vi "Write Classes.vi"(8 "error in (no error)":errorcluster, 10 "Classes":T1, 11 "Channel in":refnum<class "Channel.lvclass">) -> (0 "error out":errorcluster, 3 "Channel out":refnum<class "Channel.lvclass">)   [LabVIEW 2018, in "Channel.lvclass"]
uses:
  Channel.lvclass
  State Machine/State Machine.lvclass
  RxTx/RxTx.lvclass
  Simulated_CCD_Camera/Simulated Camera.lvclass
  Header content/Header content.lvclass
  Log File/Log File.lvclass
  Error log/Error log.lvclass
  Keywords Log File/Keywords Log File.lvclass
  Channel.lvclass/Channel.ctl
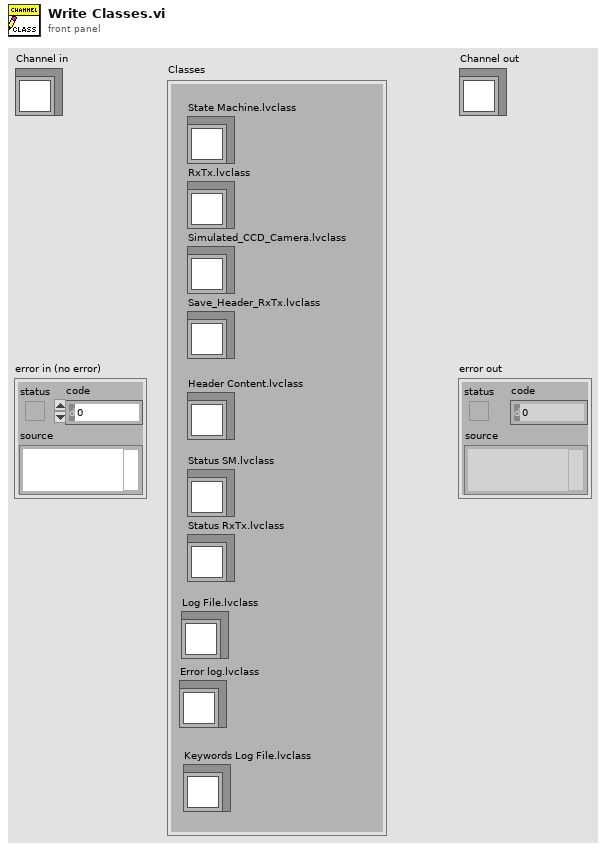
[diagram p1: front panel]
types:
  T1 = cluster{"State Machine.lvclass":refnum<class "State Machine.lvclass">, "RxTx.lvclass":refnum<class "RxTx.lvclass">, "Simulated_CCD_Camera.lvclass":refnum<class "Simulated Camera.lvclass">, "Save_Header_RxTx.lvclass":refnum<class "RxTx.lvclass">, "Header Content.lvclass":refnum<class "Header content.lvclass">, "Status SM.lvclass":refnum<class "State Machine.lvclass">, "Status RxTx.lvclass":refnum<class "RxTx.lvclass">, "Log File.lvclass":refnum<class "Log File.lvclass">, "Error log.lvclass":refnum<class "Error log.lvclass">, "Keywords Log File.lvclass":refnum<class "Keywords Log File.lvclass">}
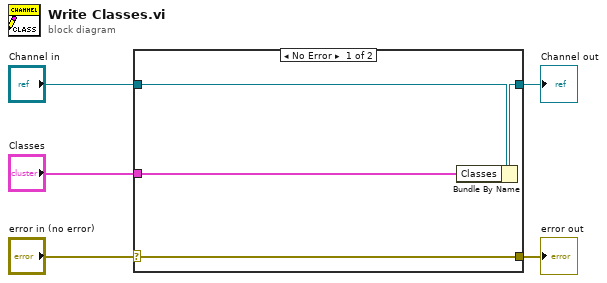
[diagram p0: block diagram]
diagram:
  n1 = case shown="No Error" "error in (no error)" {
    selector: "error in (no error)" -> [w9 w10]
    tunnel: [w9 w10] -> w4
    tunnel: [w7 w11] -> w2
    tunnel: "Channel in" -> [w8 w11]
    tunnel: "Classes" -> [w6 _]
    frame No Error {
      n2 = Bundle By Name(cluster=w8, "Classes"=w6) -> (w7:refnum<class "Channel.lvclass">)
    }
    frame Error {
    }
  }
  "error out" <- w4
  "Channel out" <- w2
